vi "Test JSON Text Comparator.vi"(11 "Test Case In":refnum<class "Comparator Tests.lvclass">) -> (0 "error out":errorcluster, 3 "Test Case Out":refnum<class "Comparator Tests.lvclass">)   [LabVIEW 2020, in "Comparator Tests.lvclass"]
uses:
  Comparator Tests.lvclass
  C:/Program Files/National Instruments/LabVIEW 2026/vi.lib/Astemes/LUnit/Test Case.lvclass
  Source/Approval Tests/JSON Comparator/JSON Comparator.lvclass
  <vilib>/Astemes/LUnit/Test Case.lvclass/Test Case.ctl
  <vilib>/Astemes/LUnit/Core/LUnit Test Case/Private/Append Fail Result.vi
  <vilib>/Astemes/LUnit/Core/LUnit Test Case/Private/Append Pass Result.vi
  <vilib>/Astemes/LUnit/Core/LUnit Test Case/Private/Run In UI.vi
  <vilib>/Utility/error.llb/Clear Errors.vi
  <vilib>/Astemes/LUnit/Test Case.lvclass
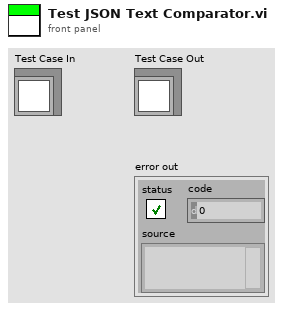
[diagram p1: front panel]
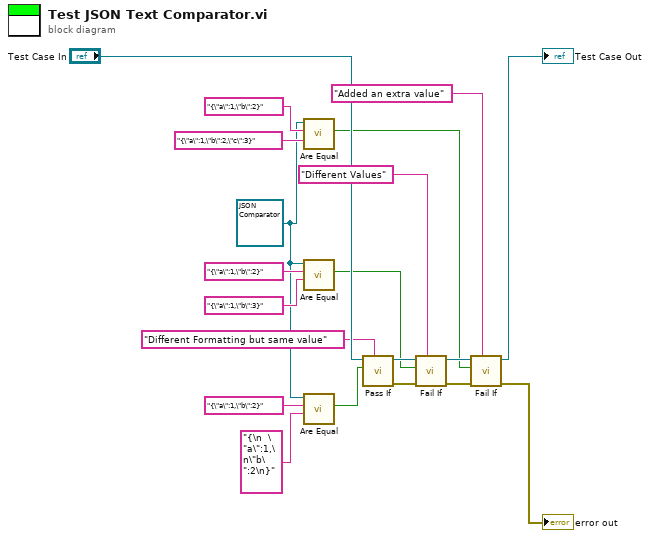
[diagram p0: block diagram]
diagram:
  w5 = refnum<class "JSON Comparator.lvclass"> refnum ("Approval Tests:JSON Comparator.lvclass")
  n1 = call-dynamic "Are Equal.vi"("Received Text"="{\"a\":1,\"b\":2,\"c\":3}" ("Approved Text"), "Approved Text"="{\"a\":1,\"b\":2}", "JSON Comparator in"=w5) -> ("Are Equal?"=w4:bool)  [unwired: 6 in, 2 out]
  n2 = call-dynamic "Are Equal.vi"("Received Text"="{\"a\":1,\"b\":3}", "Approved Text"="{\"a\":1,\"b\":2}", "JSON Comparator in"=w5) -> ("Are Equal?"=w13:bool)  [unwired: 6 in, 2 out]
  n3 = call-dynamic "Are Equal.vi"("Received Text"="{\n  \"a\":1,\n\"b\":2\n}" ("Approved Text"), "Approved Text"="{\"a\":1,\"b\":2}", "JSON Comparator in"=w5) -> ("Are Equal?"=w16:bool)  [unwired: 6 in, 2 out]
  n4 = call <vilib>:"Pass If.vi"("Description"="Different Formatting but same value", "Pass?"=w16, "LUnit Test Case In"="Test Case In") -> ("error out"=w20:errorcluster, "LUnit Test Case Out"=w15:refnum<class "Comparator Tests.lvclass">)  [unwired: 7 in]
  n5 = call <vilib>:"Fail If.vi"("Description"="Different Values", "error in (no error)"=w20, "Fail?"=w13, "LUnit Test Case In"=w15) -> ("error out"=w19:errorcluster, "LUnit Test Case Out"=w9:refnum<class "Comparator Tests.lvclass">)  [unwired: 6 in]
  n6 = call <vilib>:"Fail If.vi"("Description"="Added an extra value", "error in (no error)"=w19, "Fail?"=w4, "LUnit Test Case In"=w9) -> ("error out"=→"error out":errorcluster, "LUnit Test Case Out"=→"Test Case Out":refnum<class "Comparator Tests.lvclass">)  [unwired: 6 in]
